vi "ejer6.vi"() -> ()   [LabVIEW 2014]
uses:
  <vilib>/Analysis/Matrix/Datatypes/RealMatrix.ctl
  <vilib>/Analysis/Matrix/NI_Matrix.lvlib
panel:
  in  "Columna 1":bool
  out "Columnas":dbl[][](array[numeric])
  out "Waveform Chart":dbl[](graph)
  out "Colummna escogida":T1
  out "Columna escogida":dbl[](array[numeric])
  in  "stop":bool
  # "Salida"
  # "Gráfica"
  # "Columna 2"
  # "Filas"
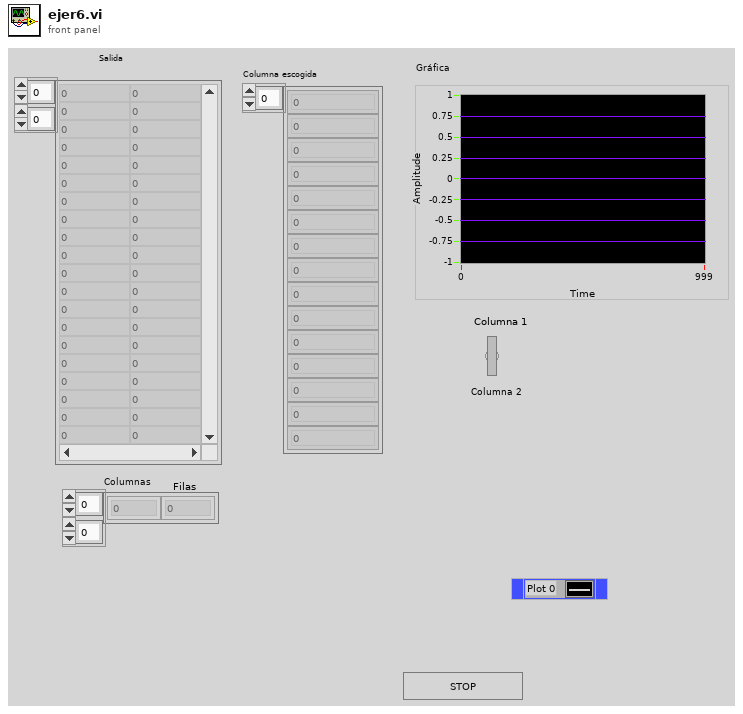
[diagram p1: front panel]
types:
  T1 = typedef "NI_Matrix.lvlib/RealMatrix.ctl" = dbl[][]
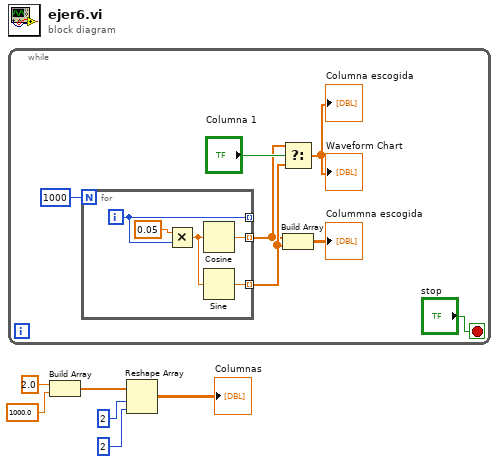
[diagram p0: block diagram]
diagram:
  n1 = while {
    stop <- "stop" stop-if-true
    n2 = for {
      N: 1000 -> [_]
      tunnel: [w14] -> w8 mode=indexing
      tunnel: [w15] -> w9 mode=indexing
      tunnel: [w17] -> _ mode=indexing
      i -> [w17]
      n3 = Multiply(x=0.05, y=w17) -> (x*y=w16:dbl)
      n4 = Cosine(x=w16) -> (cos(x)=w14:dbl)
      n5 = Sine(x=w16) -> (sin(x)=w15:dbl)
    }
    n6 = Select(t=w8, s="Columna 1", f=w9) -> (s? t:f=→"Waveform Chart" →"Columna escogida":dbl[])
    n7 = Build Array(w8, w9) -> (→"Colummna escogida":T1)
  }
  n8 = Build Array "Build Array"(2.0 ("element"), 1000.0 ("element")) -> (w4:dbl[])
  n9 = Reshape Array "Reshape Array"(w4, 2 ("dimension size"), 2 ("dimension size")) -> (→"Columnas":dbl[][])
